vi "JedanMotor_fpga_DrajverStari.vi"() -> ()   [LabVIEW 2014]
uses:
  <vilib>/rvi/Emulation/niFpgaGetClockAttributes.vi
  <vilib>/rvi/Emulation/niFpgaSctlEmulationGetInTimedLoop.vi
  <vilib>/rvi/Emulation/niFpgaEmulationReportErrorSimple.vi
  <vilib>/rvi/eio/common/nirviEmuTemplateMethod_errors.vi
  <vilib>/rvi/Emulation/niFpgaCriticalErrorInLSC.vi
  <vilib>/eio/EIONode/EIONode.xnode
panel:
  in  "stop":bool
  in  "step":sgl(knob) scale=0.0..300.0
  in  "direction":fxp<+/-,16,16>
  in  "MS3":bool
  in  "MS2":bool
  in  "MS1":bool
  # "Izaberi mod:"
  # "Izaberi smjer:"
  # "Zaustavi motor:"
  # "Izaberi brzinu motora:"
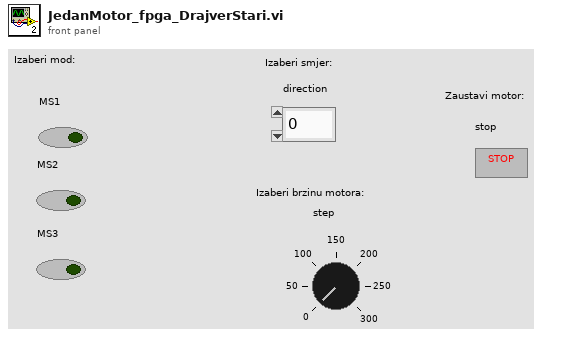
[diagram p1: front panel]
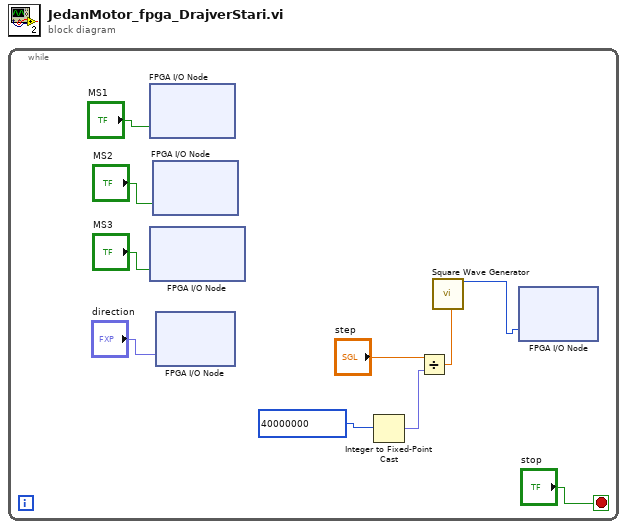
[diagram p0: block diagram]
diagram:
  n1 = while {
    stop <- "stop" stop-if-true
    n2 = xnode "FPGA I/O Node"("DIO4"="MS1") -> ()  [unwired: 1 in, 1 out]
    n3 = xnode "FPGA I/O Node"("DIO10"="MS3") -> ()  [unwired: 1 in, 1 out]
    n4 = xnode "FPGA I/O Node"("DIO7"="MS2") -> ()  [unwired: 1 in, 1 out]
    n5 = xnode "FPGA I/O Node"("AO0"="direction") -> ()  [unwired: 1 in, 1 out]
    n6 = Integer to Fixed-Point Cast(integer=40000000) -> (fixed-point=w7:fxp<+/-,32,32>)  [unwired: 1 in]
    n7 = Divide(x="step", y=w7) -> (x/y=w6:sgl)
    n8 = call "Square Wave Generator"("frequency (periods/tick)"=w6) -> ("square wave out"=w5:i32)  [unwired: 14 in]
    n9 = xnode "FPGA I/O Node"("AO1"=w5) -> ()  [unwired: 1 in, 1 out]
  }
